vi "Apply Thrust.vi"(11 "Motion in":refnum<class "Motion.lvclass">) -> (3 "Motion out":refnum<class "Motion.lvclass">)   [LabVIEW 2021, in "Motion.lvclass"]
uses:
  Motion.lvclass
  Motion.lvclass/Motion.ctl
  Vector 2D/Vector 2D.lvclass/Vector 2D.ctl
  Vector 2D/Vector 2D.lvclass
panel:
  out "Magnitude":sgl
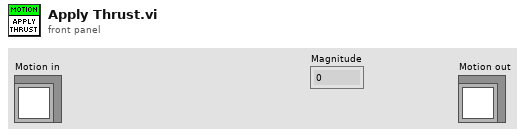
[diagram p1: front panel]
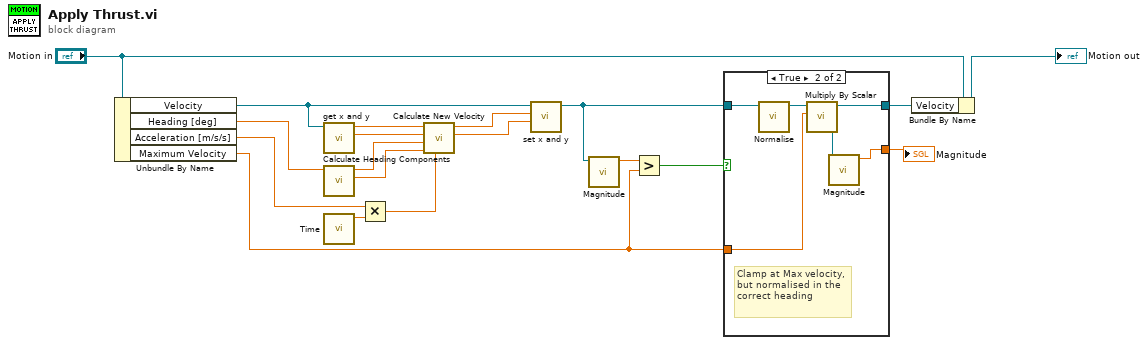
[diagram p0: block diagram]
diagram:
  n1 = Unbundle By Name("Motion in") -> ("Velocity"=w12:refnum<class "Vector 2D.lvclass">, "Heading [deg]"=w15:sgl, "Acceleration [m/s/s]"=w3:sgl, "Maximum Velocity"=w6:sgl)
  n2 = call "get x and y.vi"("Vector 2D in"=w12) -> ("y"=w10:sgl, "x"=w11:sgl)  [unwired: 9 in]
  n3 = call "Calculate Heading Components.vi"("Heading In [deg]"=w15) -> ("Sin Heading"=w19:sgl, "Cos Heading"=w18:sgl)  [unwired: 9 in]
  n4 = call "Time.vi"() -> ("Delta Time [s]"=w1:sgl)  [unwired: 10 in, 1 out]
  n5 = Multiply(x=w3, y=w1) -> (x*y=w2:sgl)
  n6 = call "Calculate New Velocity.vi"("Acceleration"=w2, "Sin Heading"=w19, "Cos Heading"=w18, "Current Velocity y"=w10, "Current Velocity x"=w11) -> ("New Velocity y"=w17:sgl, "New Velocity x"=w16:sgl)  [unwired: 5 in]
  n7 = call "set x and y.vi"("y"=w17, "x"=w16, "Vector 2D in"=w12) -> ("Vector 2D out"=w8:refnum<class "Vector 2D.lvclass">)  [unwired: 8 in]
  n8 = call "Magnitude.vi"("A"=w8) -> ("Magnitude"=w9:sgl)  [unwired: 10 in]
  n9 = Greater?(x=w9, y=w6) -> (0:w7:bool)
  n10 = case shown="True" w7 {
    tunnel: w8 -> [w20 w25]
    tunnel: w6 -> [_ w23]
    tunnel: [w20 w22] -> w5
    tunnel: [_ w21] -> w4
    frame False {
    }
    frame True {
      # "Clamp at Max velocity, but normalised in the correct heading"
      n11 = call "Normalise.vi"("Vector 2D in"=w25) -> ("Vector 2D out"=w24:refnum<class "Vector 2D.lvclass">)  [unwired: 10 in]
      n12 = call "Multiply By Scalar.vi"("x"=w23, "A"=w24) -> ("Ax"=w22:refnum<class "Vector 2D.lvclass">)  [unwired: 9 in]
      n13 = call "Magnitude.vi"("A"=w22) -> ("Magnitude"=w21:sgl)  [unwired: 10 in]
    }
  }
  "Magnitude" <- w4
  n14 = Bundle By Name(cluster="Motion in", "Velocity"=w5) -> (→"Motion out":refnum<class "Motion.lvclass">)
